vi "Get Waveform Definition.vi"(8 "error in (no error)":errorcluster, 11 "Signal Generator in":refnum<class "Signal Generator.lvclass">) -> (0 "error out":errorcluster, 2 "Waveform Definition":T1, 3 "Signal Generator out":refnum<class "Signal Generator.lvclass">)   [LabVIEW 2020, in "Signal Generator.lvlib" / "Signal Generator.lvclass"]
uses:
  Signal Generator.lvclass
  Waveform Definition.ctl
  Waveform Type.ctl
  Signal Generator.lvclass/Signal Generator.ctl
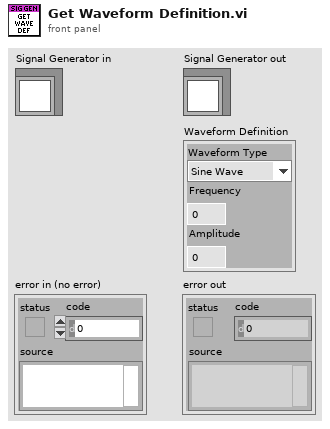
[diagram p1: front panel]
types:
  T1 = typedef "Signal Generator.lvlib/Signal Generator.lvclass/Waveform Definition.ctl" = cluster{"Waveform Type":T2, "Frequency":dbl, "Amplitude":dbl}
  T2 = typedef "Signal Generator.lvlib/Signal Generator.lvclass/Waveform Type.ctl" = enum16{"Sine Wave", "Triangle Wave", "Square Wave", "Sawtooth Wave"}
  T3 = typedef "Signal Generator.lvlib/Signal Generator.lvclass/Ref Data.ctl" = cluster{"Waveform Definition":T1}
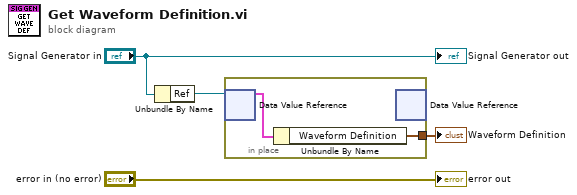
[diagram p0: block diagram]
diagram:
  n1 = Unbundle By Name("Signal Generator in") -> ("Ref"=w3:refnum<data-value>)
  n2 = in-place {
    in-place-border: [w5] -> w1
    n3 = in-place-dvr #1(w3) -> (w6:T3)  [unwired: 1 out]
    n4 = Unbundle By Name(w6) -> ("Waveform Definition"=w5:T1)
    n5 = in-place-dvr #1() -> ()  [unwired: 1 in, 2 out]
  }
  "Waveform Definition" <- w1
  "error out" <- "error in (no error)"
  "Signal Generator out" <- "Signal Generator in"
